vi "Network Setters.vi"() -> ()   [LabVIEW 2020, in "Examples.lvlib"]
uses:
  Examples.lvlib
  Network Config/Network Config.lvclass
  Protocol Config/Protocol Config.lvclass
  C:/dev/lv20CE/lv-propertybinding/Examples/Network Config/Network Config.lvclass
  PropertyBinder/Binding/Binding.lvclass/Binding.ctl
  PropertyBinder/Binding/Binding.lvclass
panel:
  out "Scheme":string
  out "Port":dbl
  out "Host":dbl
  out "error out":errorcluster
  out "Port 2":u16
  out "Host 2":string
  in  "Port":u16=8080
  in  "Host":string="192.168.42.1"
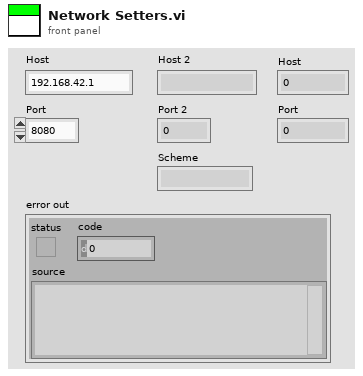
[diagram p1: front panel]
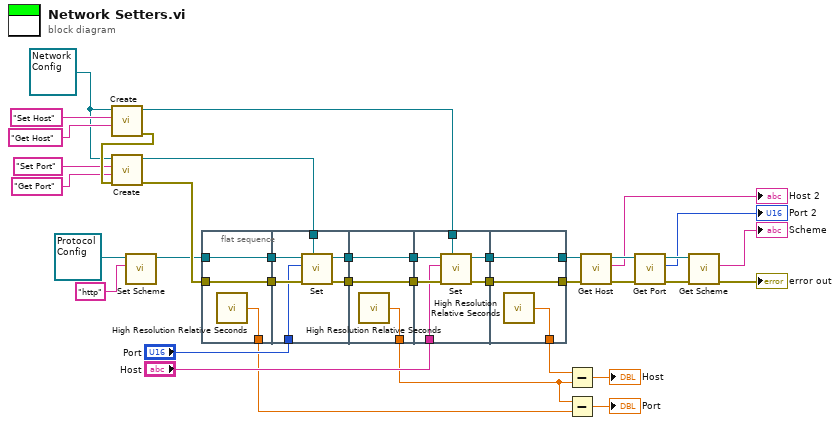
[diagram p0: block diagram]
diagram:
  w31 = refnum<class "Network Config.lvclass"> refnum ("Examples.lvlib:Network Config.lvclass")
  n1 = call "Create.vi"("Getter VI Name"="Get Host" ("Setter VI Name"), "Setter VI Name"="Set Host", "Class Type"=w31) -> ("error out"=w36:errorcluster, "Binding out"=w20:refnum<class "Binding.lvclass">)  [unwired: 7 in]
  n2 = call "Create.vi"("error in (no error)"=w36, "Getter VI Name"="Get Port" ("Setter VI Name"), "Setter VI Name"="Set Port", "Class Type"=w31) -> ("error out"=w37:errorcluster, "Binding out"=w30:refnum<class "Binding.lvclass">)  [unwired: 6 in]
  n3 = call "Set Scheme.vi"("Scheme"="http", "Protocol Config in"=refnum<class "Protocol Config.lvclass"> refnum ("Examples.lvlib:Protocol Config.lvclass")) -> ("Protocol Config out"=w7:refnum<class "Protocol Config.lvclass">)  [unwired: 8 in, 1 out]
  n4 = flat-sequence {
    tunnel: w7 -> [w39]
    tunnel: w37 -> [w40]
    tunnel: [w40] -> w26
    tunnel: [w39] -> w25
    tunnel: [w38] -> w11
    tunnel: w30 -> [w42]
    tunnel: w26 -> [w45]
    tunnel: w25 -> [w44]
    tunnel: [w46] -> w24
    tunnel: [w43] -> w23
    tunnel: "Port" -> [w41]
    tunnel: w24 -> [w49]
    tunnel: w23 -> [w48]
    tunnel: [w47] -> w12
    tunnel: [w49] -> w22
    tunnel: [w48] -> w21
    tunnel: w22 -> [w54]
    tunnel: w21 -> [w52]
    tunnel: w20 -> [w55]
    tunnel: "Host" -> [w53]
    tunnel: [w51] -> w15
    tunnel: [w50] -> w14
    tunnel: [w57] -> w17
    tunnel: [w58] -> w18
    tunnel: w15 -> [w58]
    tunnel: w14 -> [w57]
    tunnel: [w56] -> w13
    frame #0 {
      n5 = call <vilib>:"High Resolution Relative Seconds.vi"() -> ("relative seconds"=w38:dbl)
    }
    frame #1 {
      n6 = call "Set.vi"("Binding"=w42, "error in (no error)"=w45, "Value"=w41, "Class in"=w44) -> ("error out"=w46:errorcluster, "Class out"=w43:refnum<class "Protocol Config.lvclass">)  [unwired: 6 in]
    }
    frame #2 {
      n7 = call <vilib>:"High Resolution Relative Seconds.vi"() -> ("relative seconds"=w47:dbl)
    }
    frame #3 {
      n8 = call "Set.vi"("Binding"=w55, "error in (no error)"=w54, "Value"=w53, "Class in"=w52) -> ("error out"=w51:errorcluster, "Class out"=w50:refnum<class "Protocol Config.lvclass">)  [unwired: 6 in]
    }
    frame #4 {
      n9 = call <vilib>:"High Resolution Relative Seconds.vi"() -> ("relative seconds"=w56:dbl)
    }
  }
  n10 = Subtract(x=w13, y=w12) -> (x-y=→"Host":dbl)
  n11 = Subtract(x=w12, y=w11) -> (x-y=→"Port":dbl)
  n12 = call "Get Host.vi"("error in (no error)"=w18, "Network Config in"=w17) -> ("error out"=w27:errorcluster, "Host"=→"Host 2":string, "Network Config out"=w29:refnum<class "Protocol Config.lvclass">)  [unwired: 7 in]
  n13 = call "Get Port.vi"("error in (no error)"=w27, "Network Config in"=w29) -> ("error out"=w4:errorcluster, "Port"=→"Port 2":u16, "Network Config out"=w5:refnum<class "Protocol Config.lvclass">)  [unwired: 7 in]
  n14 = call "Get Scheme.vi"("error in (no error)"=w4, "Protocol Config in"=w5) -> ("error out"=→"error out":errorcluster, "Scheme"=→"Scheme":string)  [unwired: 7 in, 1 out]
